vi "RDS Read Connected.vi"(8 "error in (no error)":errorcluster, 11 "RDS Serial Instrument in":refnum<class "RDS Serial Instrument.lvclass">) -> (0 "error out":errorcluster, 2 "Connected":bool, 3 "RDS Serial Instrument out":refnum<class "RDS Serial Instrument.lvclass">)   [LabVIEW 2015, in "RDS Serial Handler.lvlib" / "RDS Serial Instrument.lvclass"]
uses:
  RDS Serial Instrument.lvclass
  RDS Serial Instrument.lvclass/RDS Serial Instrument.ctl
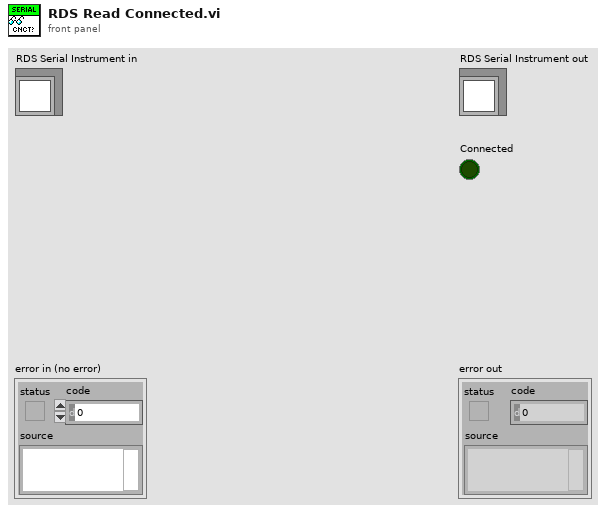
[diagram p1: front panel]
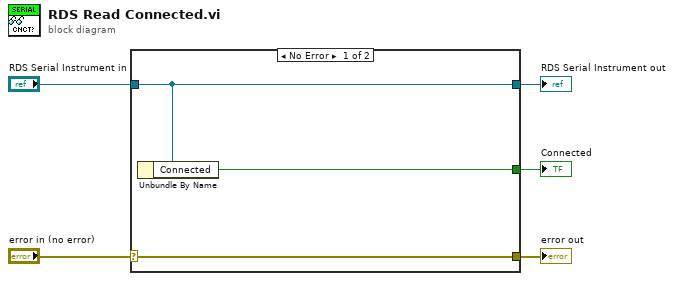
[diagram p0: block diagram]
diagram:
  n1 = case shown="No Error" "error in (no error)" {
    selector: "error in (no error)" -> [w8 w9]
    tunnel: [w8 w9] -> w4
    tunnel: [w7 w10] -> w2
    tunnel: "RDS Serial Instrument in" -> [w7 w10]
    tunnel: [w6 _] -> w1
    frame No Error {
      n2 = Unbundle By Name(w7) -> ("Connected"=w6:bool)
    }
    frame Error {
    }
  }
  "error out" <- w4
  "RDS Serial Instrument out" <- w2
  "Connected" <- w1
